vi "ConvertDDPCAGainIndex.vi"(2 "Gain (V/A)":dbl format="%#_6e", 3 "Gain (Index)":i32) -> (0 "Gain (Index)":i32, 1 "Gain (V/A)":dbl format="%#_6e")   [LabVIEW 2010]
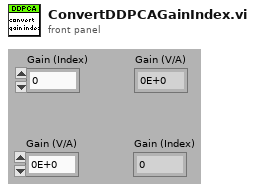
[diagram p1: front panel]
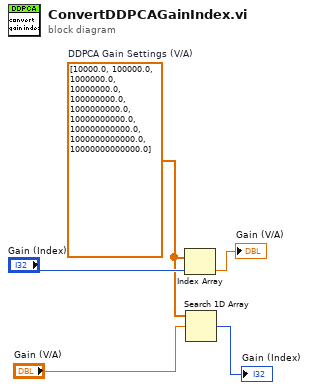
[diagram p0: block diagram]
diagram:
  w3 = dbl[] [10000.0, 100000.0, 1000000.0, 10000000.0, 100000000.0, 1000000000.0, 10000000000.0, 100000000000.0, 1000000000000.0, 10000000000000.0]  # DDPCA Gain Settings (V/A)
  n1 = Index Array(array=w3, index="Gain (Index)") -> (element=→"Gain (V/A)":dbl)
  n2 = Search 1D Array(1D array=w3, element="Gain (V/A)") -> (index of element=→"Gain (Index)":i32)  [unwired: 1 in]
